vi "Write heartbeat.vi"(8 "error in (no error)":errorcluster, 10 "heartbeat":T1={"lastUpdateTime"=0.0, "period"=1.0, "timeout"=0.0, "lastSuccesfulUpdateTime"=0.0}, 11 "deviceHeartbeat in":refnum<class "deviceHeartbeat.lvclass">) -> (0 "error out":errorcluster, 3 "deviceHeartbeat out":refnum<class "deviceHeartbeat.lvclass">)   [LabVIEW 2016, in "deviceHeartbeat.lvclass"]
uses:
  deviceHeartbeat.lvclass
  typedefs/heartbeat.ctl
  deviceHeartbeat.lvclass/deviceHeartbeat.ctl
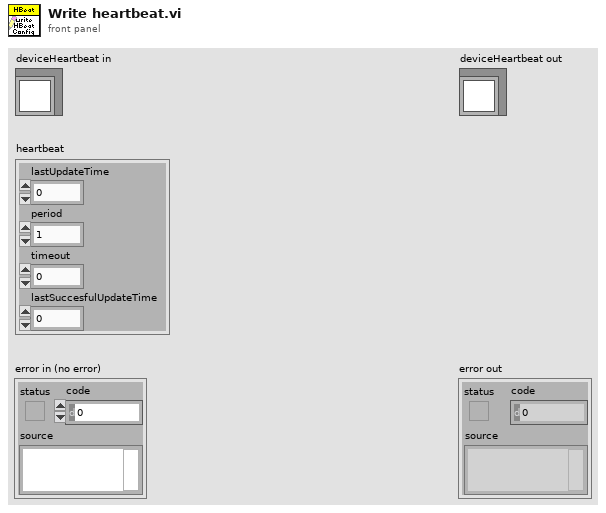
[diagram p1: front panel]
types:
  T1 = typedef "heartbeat.ctl" = cluster{"lastUpdateTime":dbl, "period":dbl, "timeout":dbl, "lastSuccesfulUpdateTime":dbl}
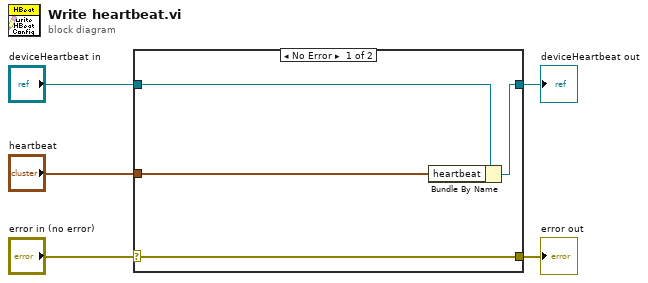
[diagram p0: block diagram]
diagram:
  n1 = case shown="No Error" "error in (no error)" {
    selector: "error in (no error)" -> [w9 w10]
    tunnel: [w9 w10] -> w4
    tunnel: [w7 w11] -> w2
    tunnel: "deviceHeartbeat in" -> [w8 w11]
    tunnel: "heartbeat" -> [w6 _]
    frame No Error {
      n2 = Bundle By Name(cluster=w8, "heartbeat"=w6) -> (w7:refnum<class "deviceHeartbeat.lvclass">)
    }
    frame Error {
    }
  }
  "error out" <- w4
  "deviceHeartbeat out" <- w2
